vi "Toggle.vi"(11 "Input":bool) -> (3 "Output":bool)   [LabVIEW 2013]
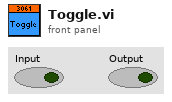
[diagram p1: front panel]
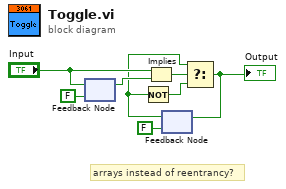
[diagram p0: block diagram]
diagram:
  # "arrays instead of reentrancy?"
  n1 = feedback #1(FALSE) -> (w6:bool)
  n2 = feedback-in #1("Input") -> ()
  n3 = Implies(1:w6, 2:"Input") -> (0:w1:bool)
  n4 = feedback #2(FALSE) -> (w4:bool)
  n5 = Not(x=w4) -> (.not. x?=w2:bool)
  n6 = Select(t=w4, s=w1, f=w2) -> (s? t:f=w8:bool)
  "Output" <- w8
  n7 = feedback-in #2(w8) -> ()
